vi "errortest.vi"(11 "Error Code":i32=7) -> (3 "Error Text":string)   [LabVIEW 2021, in "error.lvlib"]
uses:
  error.lvlib
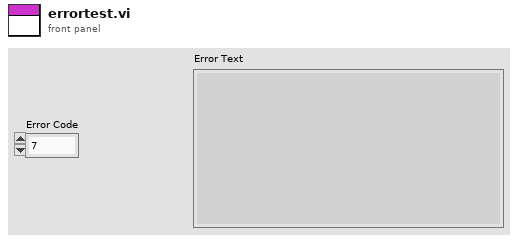
[diagram p1: front panel]
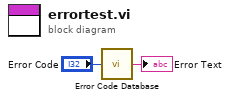
[diagram p0: block diagram]
diagram:
  n1 = call <vilib>:"Error Code Database.vi"("Error Code"="Error Code") -> ("Error Text"=→"Error Text":string)
